vi "Enable disable controls.vi"(0 "Enable reference":refnum<vi>[](array[refnum]), 5 "Disable reference":refnum<vi>[](array[refnum]), 11 "Error in":errorcluster) -> (15 "Error out":errorcluster)   [LabVIEW 2020, in "Custom Sort Function.lvlib"]
uses:
  Libraries/Custom Sort Function.lvlib
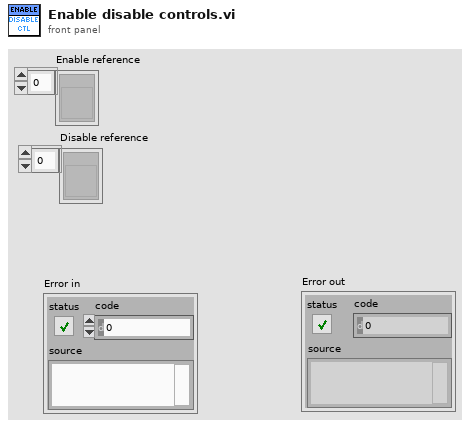
[diagram p1: front panel]
types:
  T1 = enum8{"Enabled", "Disabled", "Disabled and Grayed Out"}
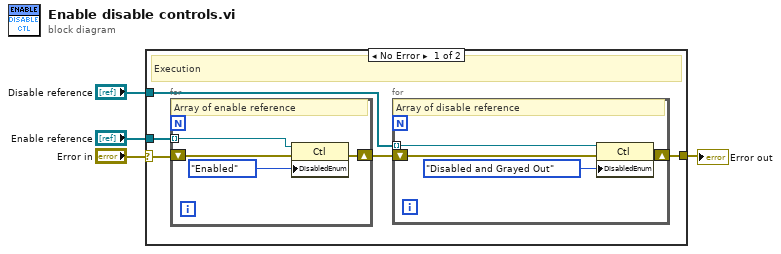
[diagram p0: block diagram]
diagram:
  n1 = case shown="No Error" "Error in" {
    selector: "Error in" -> [w5 w18]
    tunnel: [w8 w18] -> w4
    tunnel: "Disable reference" -> [w7 _]
    tunnel: "Enable reference" -> [w6 _]
    frame No Error {
      # "Execution"
      n2 = for {
        shift-right: [w13] -> w9
        shift-left: w5 -> [w12]
        tunnel: w6 -> [w10] mode=indexing
        # "Array of enable reference"
        n3 = property class="Ctl"(reference=w10, error in=w12, "DisabledEnum"=T1."Enabled" ("Disabled")) -> (error out=w13:errorcluster)  [unwired: 1 out]
      }
      n4 = for {
        shift-right: [w15] -> w8
        shift-left: w9 -> [w16]
        tunnel: w7 -> [w14] mode=indexing
        # "Array of disable reference"
        n5 = property class="Ctl"(reference=w14, error in=w16, "DisabledEnum"=T1."Disabled and Grayed Out" ("Disabled")) -> (error out=w15:errorcluster)  [unwired: 1 out]
      }
    }
    frame Error {
      # "Terminate if error"
    }
  }
  "Error out" <- w4
